vi "opencvSegmentConvertCoordinates-multiFrames.vi"(1 "sizex":u16=256, 2 "NeuronN":u16[](array[numeric]), 3 "NeuronXY":u16[][](array[numeric])) -> (0 "XY":u16[][][](array[numeric]))   [LabVIEW 2017]
panel:
  # "Converts the coordinates from the 1D representation of the image to XY."
  # "NeuronXY[frame,neuron]"
  # "XY[frame,neuron,coordinate]"
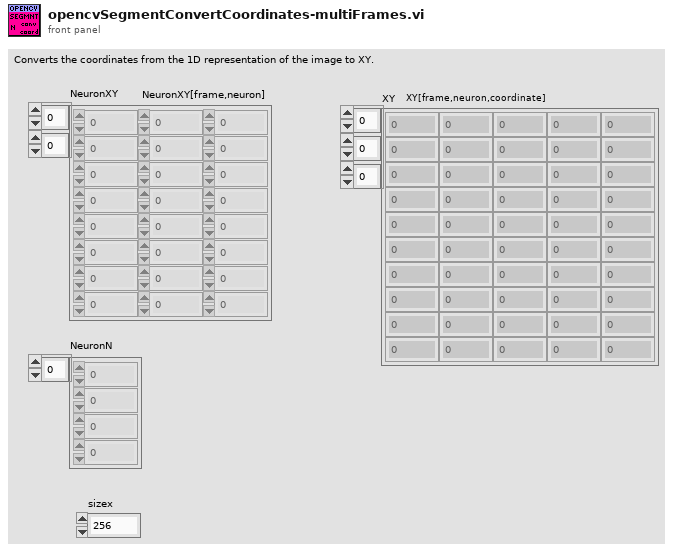
[diagram p1: front panel]
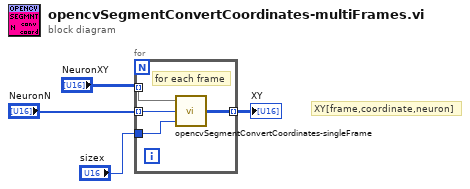
[diagram p0: block diagram]
diagram:
  # "XY[frame,coordinate,neuron]"
  n1 = for {
    tunnel: "NeuronXY" -> [w7] mode=indexing
    tunnel: "sizex" -> [w8]
    tunnel: [w6] -> w2 mode=indexing
    tunnel: "NeuronN" -> [w5] mode=indexing
    # "for each frame"
    n2 = call "opencvSegmentConvertCoordinates-singleFrame.vi"("sizex2"=w8, "NeuronN"=w5, "NeuronXY"=w7) -> ("XY"=w6:u16[][])
  }
  "XY" <- w2
